vi "_Open Help in Default Browser.vi"(8 "error in (no error)":errorcluster, 11 "name or relative path":string) -> (0 "error out":errorcluster)   [LabVIEW 2017]
uses:
  <vilib>/Platform/browser.llb/Open URL in Default Browser (path).vi
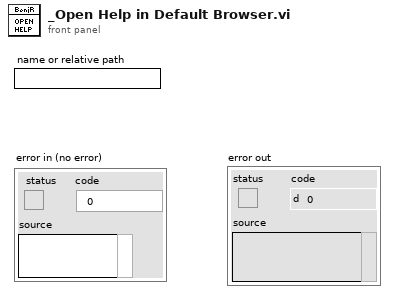
[diagram p1: front panel]
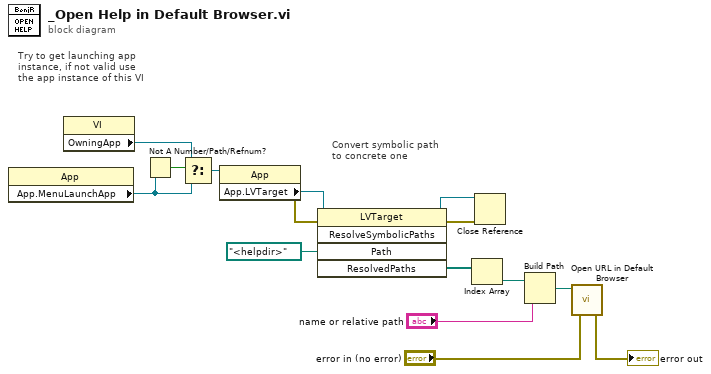
[diagram p0: block diagram]
diagram:
  # "Convert symbolic path\nto concrete one"
  # "Try to get launching app\ninstance, if not valid use\nthe app instance of this VI"
  n1 = property class="App"() -> ("App.MenuLaunchApp"=w3:refnum<vi>)  [unwired: 2 in, 2 out]
  n2 = property class="VI"() -> ("OwningApp"=w4:refnum<vi>)  [unwired: 2 in, 2 out]
  n3 = Not A Number/Path/Refnum?(number/path/refnum=w3) -> (NaN/Path/Refnum?=w5:bool)
  n4 = Select(t=w4, s=w5, f=w3) -> (s? t:f=w2:refnum<vi>)
  n5 = property class="App"(reference=w2) -> (error out=w10:errorcluster, "App.LVTarget"=w9:refnum<vi>)  [unwired: 1 in, 1 out]
  n6 = invoke class="LVTarget" method="ResolveSymbolicPaths"(reference=w9, error in=w10, "Path"=path "<helpdir>" ("base path")) -> (reference out=w6:refnum<vi>, error out=w7:errorcluster, "ResolvedPaths"=w11:path[])  [unwired: 2 in, 2 out]
  n7 = Index Array(array=w11) -> (element=w1:path)  [unwired: 1 in]
  n8 = Close Reference(reference=w6, error in (no error)=w7) -> ()  [unwired: 1 out]
  n9 = Build Path(base path=w1, name or relative path="name or relative path") -> (appended path=w15:path)
  n10 = call-poly <vilib>:"Open URL in Default Browser.vi"("error in (no error)"="error in (no error)", "path"=w15) -> ("error out"=→"error out":errorcluster)  [unwired: 4 in, 1 out]
